vi "BuildSpec2.vi"() -> ()   [LabVIEW 2026, in "BuildSpecLib.lvlib"]
uses:
  BuildSpecLib.lvlib
panel:
  out "x+y":dbl
  in  "x":dbl
  in  "y":dbl
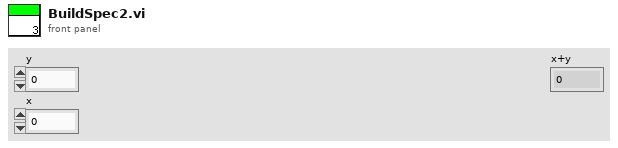
[diagram p1: front panel]
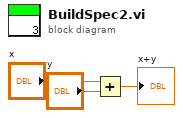
[diagram p0: block diagram]
diagram:
  n1 = Add(x="x", y="y") -> (x+y=→"x+y":dbl)
